vi "My Arithmetic Average.vi"() -> ()   [LabVIEW 2020]
panel:
  out "Arithmetic Average":dbl
  in  "3rd Number":dbl
  in  "2nd Number":dbl
  in  "1st Number":dbl
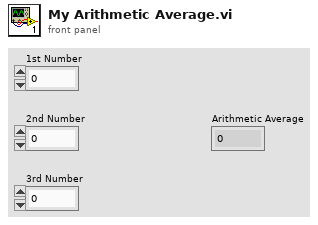
[diagram p1: front panel]
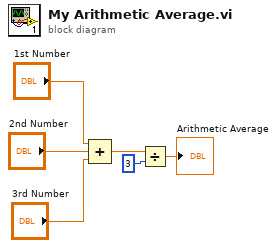
[diagram p0: block diagram]
diagram:
  n1 = Compound Arithmetic op=ADD("1st Number", "2nd Number", "3rd Number") -> (w3:dbl)
  n2 = Divide(x=w3, y=3) -> (x/y=→"Arithmetic Average":dbl)
